vi "Get Status.vi"(8 "error in (no error)":errorcluster, 11 "Scanner.lvclass in":refnum<class "Scanner.lvclass">) -> (0 "error out":errorcluster, 2 "Status":string, 3 "Scanner.lvclass out":refnum<class "Scanner.lvclass">)   [LabVIEW 2017, in "Scanner.lvclass"]
uses:
  Scanner.lvclass
  Scanner.lvclass/Scanner.ctl
  Global/File Locations.vi
  Instruments/Utility Classes/Scannable/Scannable.lvclass
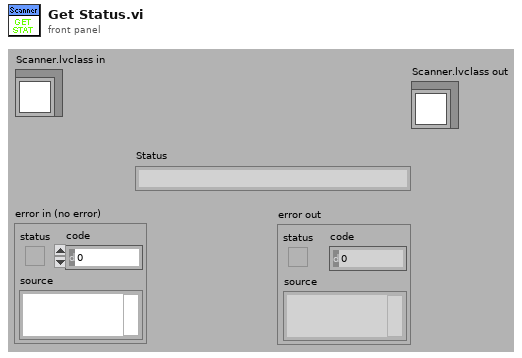
[diagram p1: front panel]
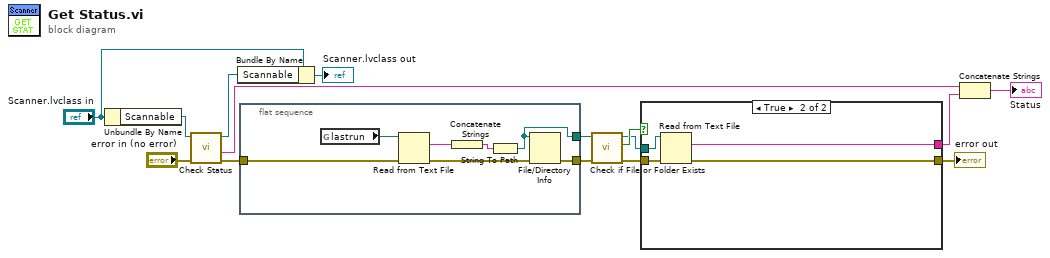
[diagram p0: block diagram]
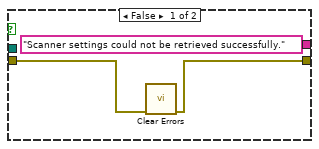
[diagram p2: hidden frame]
diagram:
  n1 = Unbundle By Name("Scanner.lvclass in") -> ("Scannable"=w13:refnum<class "Scannable.lvclass">)
  n2 = call-dynamic "Check Status.vi"("error in (no error)"="error in (no error)", "Instrument in"=w13) -> ("error out"=w7:errorcluster, "Status"=w15:string, "Instrument out"=w11:refnum<class "Scannable.lvclass">)  [unwired: 6 in, 1 out]
  n3 = Bundle By Name(cluster="Scanner.lvclass in", "Scannable"=w11) -> (→"Scanner.lvclass out":refnum<class "Scanner.lvclass">)
  n4 = flat-sequence {
    tunnel: [w22] -> w8
    tunnel: [w18] -> w9
    tunnel: w7 -> [w17]
    frame #0 {
      n5 = global read "File Locations.vi" "lastrun"() -> (w20:path)
      n6 = Read from Text File(file (use dialog)=w20, error in=w17) -> (text=w21:string, error out=w19:errorcluster)  [unwired: 4 out]
      n7 = Concatenate Strings(w21) -> (w16:string)
      n8 = String To Path(string=w16) -> (path=w22:path)
      n9 = File/Directory Info(path=w22, error in=w19) -> (error out=w18:errorcluster)  [unwired: 6 out]
    }
  }
  n10 = call <vilib>:"Check if File or Folder Exists.vi"("error in (no error)"=w9, "path"=w8) -> ("error out"=w4:errorcluster, "file or folder exists?"=w6:bool, "dup path"=w5:path)  [unwired: 7 in]
  n11 = case shown="True" w6 {
    tunnel: w5 -> [_ w29]
    tunnel: w4 -> [w24 w28]
    tunnel: ["Scanner settings could not be retrieved successfully." w27] -> w2
    tunnel: [w23 w26] -> w1
    frame False {
      n12 = call <vilib>:"Clear Errors.vi"("error in (no error)"=w24) -> ("error out"=w23:errorcluster)  [unwired: 5 in, 1 out]
    }
    frame True {
      n13 = Read from Text File(file (use dialog)=w29, error in=w28) -> (text=w27:string, error out=w26:errorcluster)  [unwired: 2 in, 2 out]
    }
  }
  "error out" <- w1
  n14 = Concatenate Strings(w15, w2) -> (→"Status":string)
